vi "TDMS_Channel_Write.vi"(10 "Data":dbl, 11 "TDMS Channel Info in":T1={"TDMS Data"={"Group/CMD"=-2, "Channel"=-2, "Data"=0.0}, "TDMS RT FIFO"=refnum}) -> (3 "TDMS Channel Info out":T1={"TDMS Data"={"Group/CMD"=-2, "Channel"=-2, "Data"=0.0}, "TDMS RT FIFO"=refnum})   [LabVIEW 2015]
uses:
  <userlib>/836-Library/System/TDMSv2/TDMS_Channel_Info.ctl
  <userlib>/836-Library/System/TDMSv2/TDMS_RT_FIFO_Packet.ctl
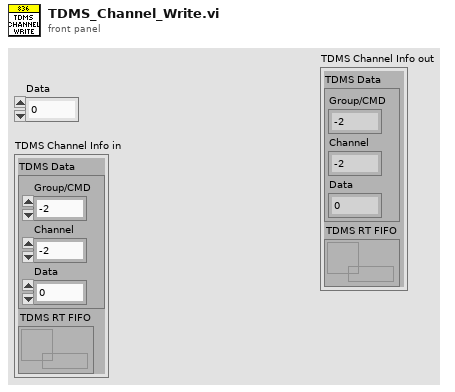
[diagram p1: front panel]
types:
  T1 = typedef "TDMS_Channel_Info.ctl" = cluster{"TDMS Data":T2, "TDMS RT FIFO":refnum<k33>}
  T2 = typedef "TDMS_RT_FIFO_Packet.ctl" = cluster{"Group/CMD":i32, "Channel":i32, "Data":dbl}
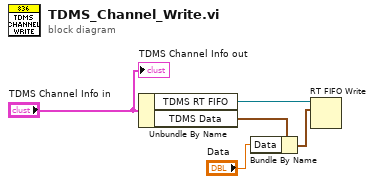
[diagram p0: block diagram]
diagram:
  n1 = Unbundle By Name("TDMS Channel Info in") -> ("TDMS RT FIFO"=w2:refnum<k33>, "TDMS Data"=w3:T2)
  n2 = Bundle By Name(cluster=w3, "Data"="Data") -> (w5:T2)
  n3 = RT FIFO Write(0:w2, 1:w5) -> ()  [unwired: 3 in, 4 out]
  "TDMS Channel Info out" <- "TDMS Channel Info in"
